vi "Set_Start_Method_Info.vi"(8 "expId":string) -> (3 "String":string)   [LabVIEW 2014]
doc: "Sets the JSON-RPC 2.0 message for the 'start' method"
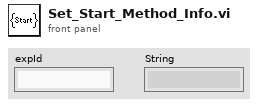
[diagram p1: front panel]
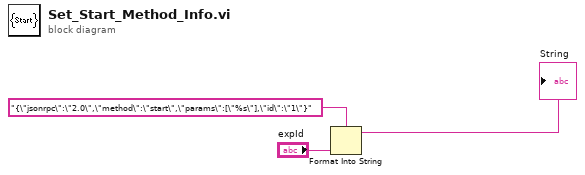
[diagram p0: block diagram]
diagram:
  n1 = Format Into String(format string="{\"jsonrpc\":\"2.0\",\"method\":\"start\",\"params\":[\"%s\"],\"id\":\"1\"}" ("input string"), "expId") -> (resulting string=→"String":string)  [unwired: 2 in, 1 out]
